vi "Sub_Python_cmd_eigh.vi"(10 "Stiff":dbl[][](array[numeric])=array80x80[6400 elements], 11 "Mass":dbl[][](array[numeric])) -> (2 "Eigenvectors":dbl[][](array[numeric]), 3 "Eigenvalues":dbl[](array[numeric]))   [LabVIEW 2021]
uses:
  <vilib>/Utility/file.llb/Write Delimited Spreadsheet (DBL).vi
  <vilib>/Utility/file.llb/Read Delimited Spreadsheet (DBL).vi
panel:
  out "Elapsed time":dbl=0.5790897820043028
  out "standard error":string
  out "standard output":string
  # "This VI is necesary as the installed version of LabView is 32 bit and anaconda installation is 64 bit making a python node call not possible without moving the chasis onto a secure network. The native LabView Eigensolver does not work with the Secular Equation Solver developed for lemp due to how each solver scales its mode shapes.  This can be replaced if the scaling between the two could be reconciled. Regardless, the task must only be implemented once for LEMP on initailization and so it is a Low Priority optimization despite the task taking  ~ 0.6 sec for 40 nodes. \n\nDocumentation was too scarce for me to reconcile the issue with the Labview Eigenvector scaling versus Scipy's Eigh.\n              - Alexander Vereen AFRL Summer scholars 2022"
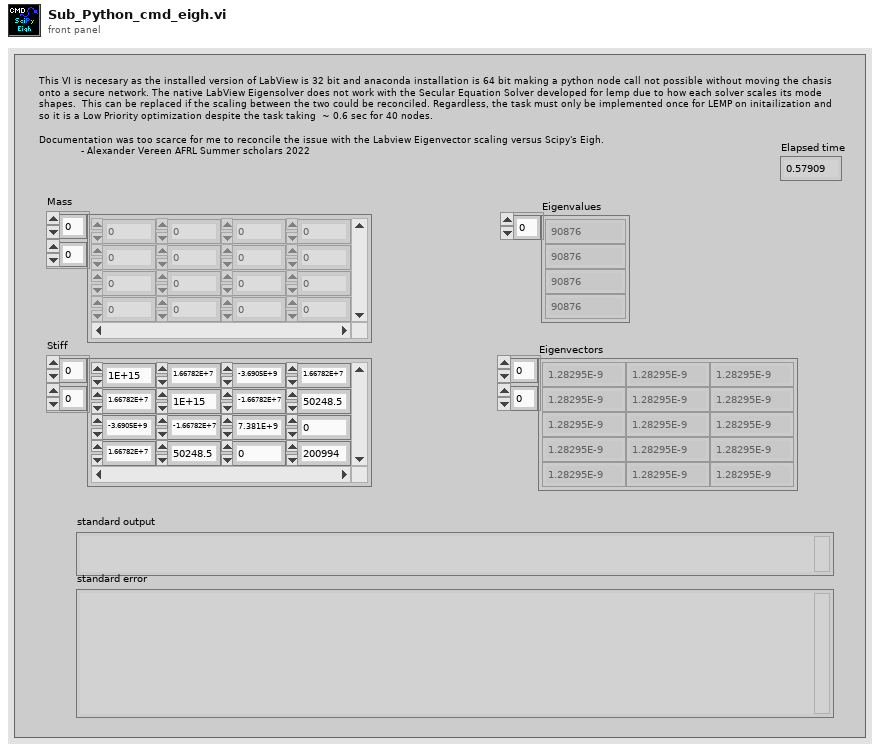
[diagram p1: front panel]
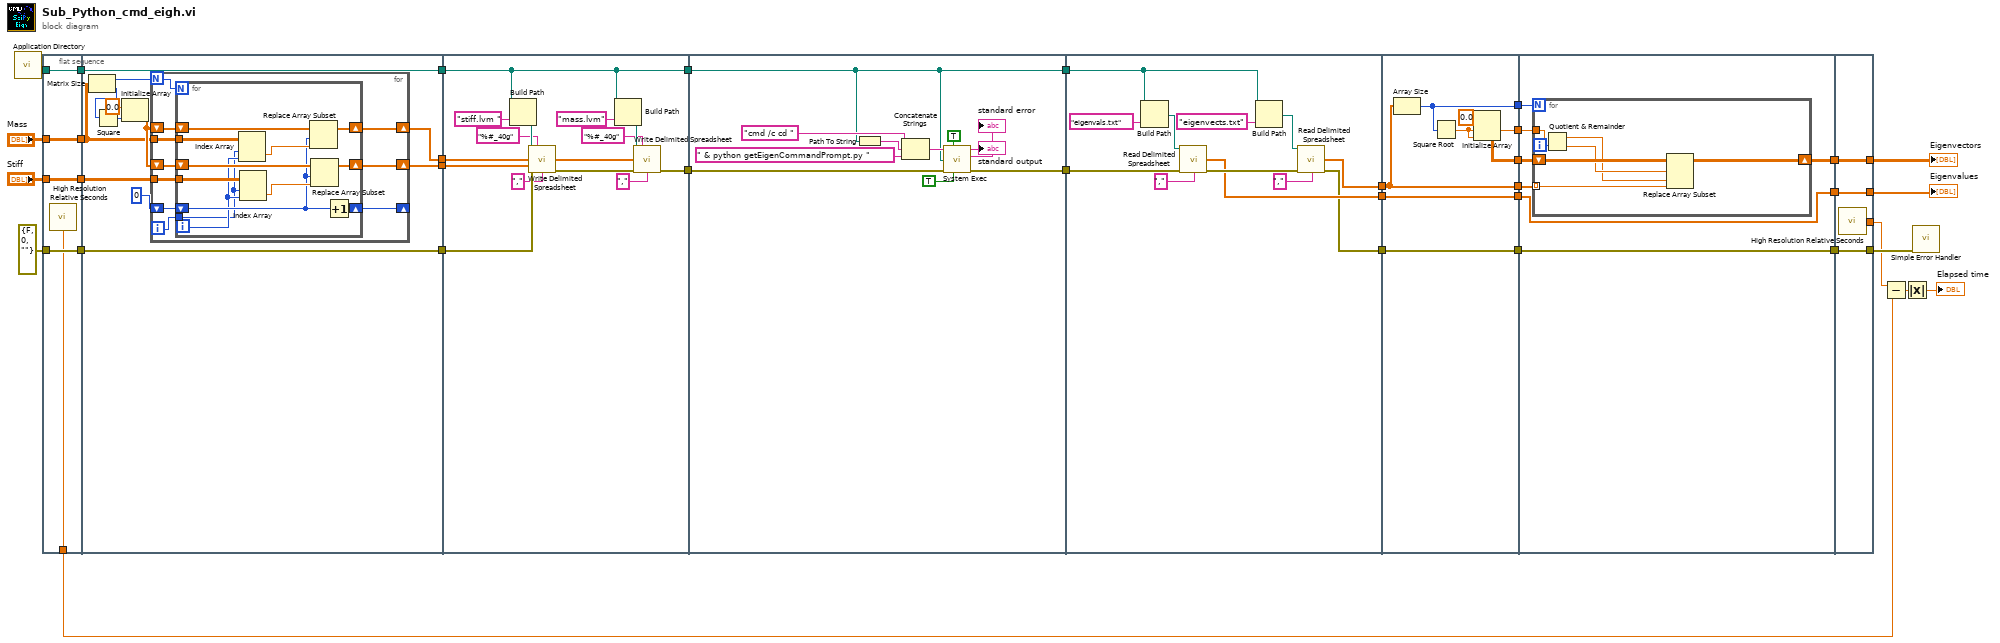
[diagram p0: block diagram]
diagram:
  n1 = call <vilib>:"Application Directory.vi"() -> ("Application Directory"=w32:path)
  n2 = flat-sequence {
    tunnel: errorcluster {"status"=FALSE, "code"=0, "source"=""} ("error in (no error)") -> [w37]
    tunnel: w32 -> [w38]
    tunnel: "Mass" -> [w39]
    tunnel: "Stiff" -> [w40]
    tunnel: [w40] -> w11
    tunnel: [w39] -> w10
    tunnel: [w38] -> w9
    tunnel: [w37] -> w8
    tunnel: [w36] -> w3
    tunnel: [w45] -> w20
    tunnel: [w44] -> w19
    tunnel: [w52] -> w18
    tunnel: [w51] -> w17
    tunnel: w11 -> [w42]
    tunnel: w10 -> [w43]
    tunnel: w9 -> [w52]
    tunnel: w8 -> [w51]
    tunnel: [w87] -> w33
    tunnel: [w85] -> w30
    tunnel: w20 -> [w76]
    tunnel: w19 -> [w75]
    tunnel: w18 -> [w85]
    tunnel: w17 -> [w86]
    tunnel: w33 -> [w98]
    tunnel: [w97] -> w13
    tunnel: w30 -> [w91]
    tunnel: [w91] -> w12
    tunnel: w13 -> [w111]
    tunnel: w12 -> [w109]
    tunnel: [w104] -> w29
    tunnel: [w103] -> w28
    tunnel: [w100] -> w16
    tunnel: w29 -> [w113]
    tunnel: w28 -> [w115]
    tunnel: [w118] -> w27
    tunnel: [w116] -> w26
    tunnel: [w115] -> w25
    tunnel: [w114] -> w24
    tunnel: [w113] -> w23
    tunnel: w16 -> [w112]
    tunnel: [w112] -> w15
    tunnel: w27 -> [w125]
    tunnel: w26 -> [w124]
    tunnel: w25 -> [w123]
    tunnel: w24 -> [w122]
    tunnel: w23 -> [w120]
    tunnel: w15 -> [w119]
    tunnel: [w121] -> w7
    tunnel: [w120] -> w6
    tunnel: [w119] -> w5
    tunnel: w7 -> [w136]
    tunnel: w6 -> [w135]
    tunnel: w5 -> [w134]
    tunnel: [w136] -> w21
    tunnel: [w135] -> w22
    tunnel: [w134] -> w14
    tunnel: [w133] -> w4
    frame #0 {
      n3 = call <vilib>:"High Resolution Relative Seconds.vi"() -> ("relative seconds"=w36:dbl)
    }
    frame #1 {
      n4 = Matrix Size(0:w43) -> (1:w50:i32, 2:w48:i32)
      n5 = Square(x=w48) -> (x^2=w49:i32)
      n6 = Initialize Array(0.0 ("element"), w49) -> (w46:dbl[])
      n7 = for {
        N: w50 -> [w54]
        shift-right: [w59] -> w44
        shift-left: w46 -> [w60]
        shift-right: [w61] -> w45
        shift-left: w46 -> [w62]
        tunnel: w43 -> [w57]
        tunnel: w42 -> [w56]
        shift-right: [w53] -> _
        shift-left: u32 0 -> [w55]
        i -> [w58]
        n8 = for {
          N: w54 -> [_]
          tunnel: w58 -> [w63]
          tunnel: w57 -> [w68]
          tunnel: w56 -> [w67]
          shift-right: [w66] -> w53
          shift-left: w55 -> [w65]
          shift-right: [w71] -> w59
          shift-left: w60 -> [w72]
          shift-right: [w73] -> w61
          shift-left: w62 -> [w74]
          i -> [w64]
          n9 = Index Array(array=w68, index (row)=w63, index (col)=w64) -> (element=w70:dbl)
          n10 = Index Array(array=w67, index (row)=w63, index (col)=w64) -> (element=w69:dbl)
          n11 = Replace Array Subset(array=w72, new element=w70, index=w65) -> (w71:dbl[])
          n12 = Replace Array Subset(array=w74, new element=w69, index=w65) -> (w73:dbl[])
          n13 = Increment(x=w65) -> (x+1=w66:u32)
        }
      }
    }
    frame #2 {
      n14 = Build Path(base path=w85, name or relative path="stiff.lvm ") -> (appended path=w83:path)
      n15 = call-poly <vilib>:"Write Delimited Spreadsheet.vi"("file path (dialog if empty)"=w83, "format (%.3f)"="%#_40g", "1D data"=w76, "error in (no error)"=w86, "delimiter (\\t)"="," ("delimiter (\\t)")) -> ("error out"=w88:errorcluster)  [unwired: 9 in, 1 out]
      n16 = Build Path(base path=w85, name or relative path="mass.lvm") -> (appended path=w84:path)
      n17 = call-poly <vilib>:"Write Delimited Spreadsheet.vi"("file path (dialog if empty)"=w84, "format (%.3f)"="%#_40g", "1D data"=w75, "error in (no error)"=w88, "delimiter (\\t)"="," ("delimiter (\\t)")) -> ("error out"=w87:errorcluster)  [unwired: 9 in, 1 out]
    }
    frame #3 {
      n18 = Path To String(path=w91) -> (string=w90:string)
      n19 = Concatenate Strings("cmd /c cd " ("command line"), w90, " & python getEigenCommandPrompt.py " ("standard input")) -> (w92:string)
      n20 = call <vilib>:"System Exec.vi"("run minimized? (F)"=TRUE, "wait until completion? (T)"=TRUE, "error in (no error)"=w98, "working directory"=w91, "command line"=w92) -> ("error out"=w97:errorcluster, "standard error"=→"standard error":string, "standard output"=→"standard output":string)  [unwired: 3 in, 1 out]
    }
    frame #4 {
      n21 = Build Path(base path=w109, name or relative path="eigenvals.txt") -> (appended path=w108:path)
      n22 = call-poly <vilib>:"Read Delimited Spreadsheet.vi"("file path (dialog if empty)"=w108, "error in (no error)"=w111, "delimiter (\\t)"="," ("delimiter (\\t)")) -> ("first row"=w104:dbl[], "error out"=w110:errorcluster)  [unwired: 7 in, 4 out]
      n23 = Build Path(base path=w109, name or relative path="eigenvects.txt") -> (appended path=w107:path)
      n24 = call-poly <vilib>:"Read Delimited Spreadsheet.vi"("file path (dialog if empty)"=w107, "error in (no error)"=w110, "delimiter (\\t)"="," ("delimiter (\\t)")) -> ("first row"=w103:dbl[], "error out"=w100:errorcluster)  [unwired: 7 in, 4 out]
    }
    frame #5 {
      n25 = Array Size(array=w115) -> (size(s)=w118:i32)
      n26 = Square Root(x=w118) -> (sqrt(x)=w114:dbl)
      n27 = Initialize Array(0.0 ("element"), w114, w114) -> (w116:dbl[][])
    }
    frame #6 {
      n28 = for {
        N: w125 -> [_]
        shift-right: [w128] -> w121
        shift-left: w124 -> [w131]
        tunnel: w123 -> [w130] mode=indexing
        tunnel: w122 -> [w127]
        i -> [w132]
        n29 = Quotient & Remainder(x=w132, y=w127) -> (x-y*floor(x/y)=w126:dbl, floor(x/y)=w129:dbl)
        n30 = Replace Array Subset(array=w131, new element=w130, index (row)=w129, index (col)=w126) -> (w128:dbl[][])
      }
    }
    frame #7 {
      n31 = call <vilib>:"High Resolution Relative Seconds.vi"() -> ("relative seconds"=w133:dbl)
    }
  }
  n32 = Subtract(x=w4, y=w3) -> (x-y=w2:dbl)
  n33 = Absolute Value(x=w2) -> (abs(x)=→"Elapsed time":dbl)
  n34 = call <vilib>:"Simple Error Handler.vi"("error in (no error)"=w14) -> ()  [unwired: 4 in, 5 out]
  "Eigenvalues" <- w22
  "Eigenvectors" <- w21
